vi "__PW_1ch.vi"(6 "Wait(ms)":i32=800, 8 "Ch（A,B,C,D）":string="A", 9 "A(A)":dbl=0.9, 10 "V(V)":dbl, 11 "GPIB":string="3") -> (1 "Amoni":dbl, 2 "Vmoni":dbl=0.05)   [LabVIEW 2017]
panel:
  out "文字列":string="VA0.00,AA0.90"
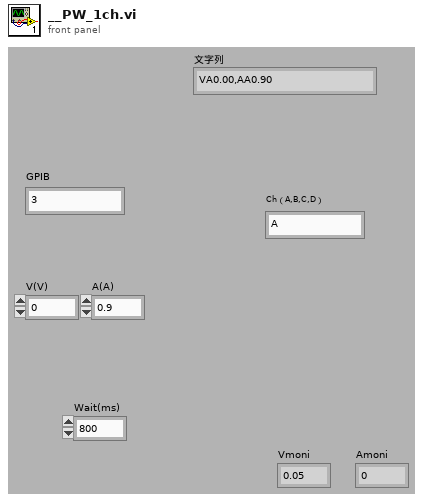
[diagram p1: front panel]
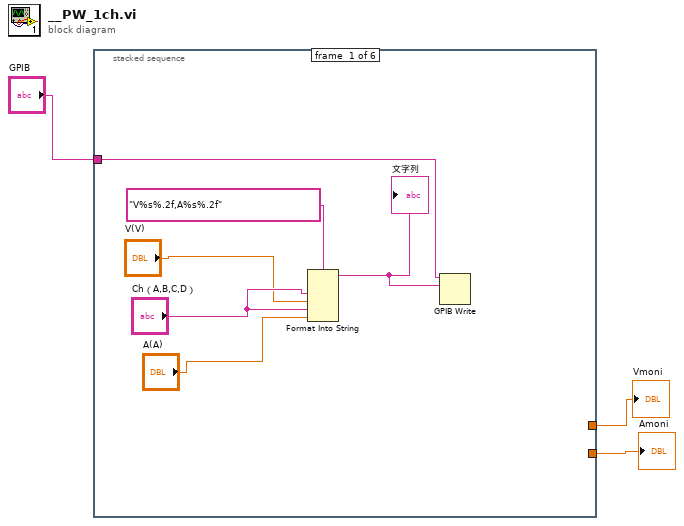
[diagram p0: block diagram]
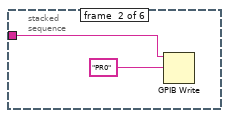
[diagram p2: hidden frame]
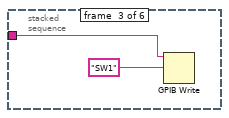
[diagram p3: hidden frame]
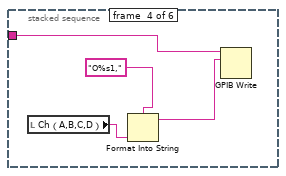
[diagram p4: hidden frame]
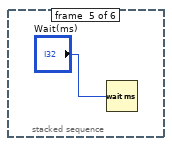
[diagram p5: hidden frame]
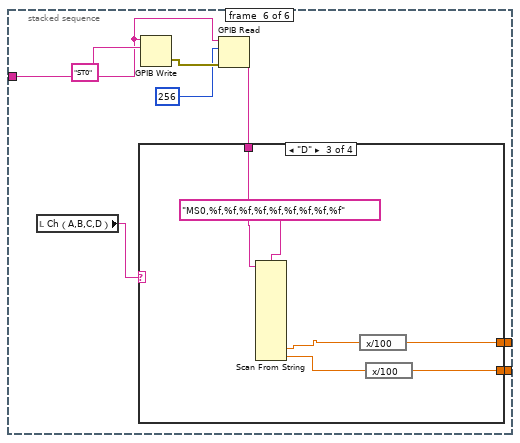
[diagram p6: hidden frame]
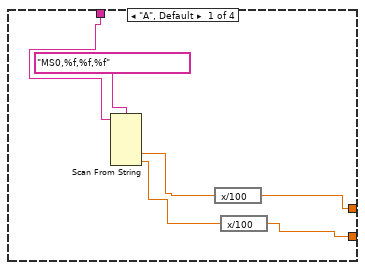
[diagram p7: hidden frame]
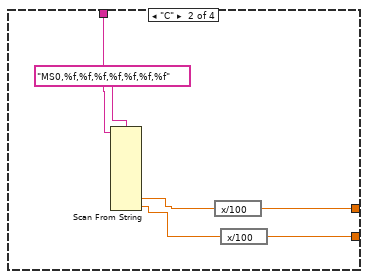
[diagram p8: hidden frame]
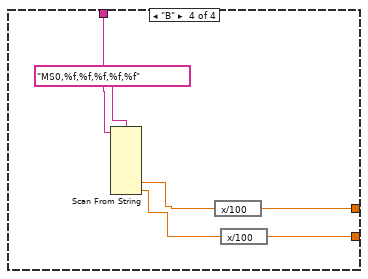
[diagram p9: hidden frame]
diagram:
  n1 = stacked-sequence {
    tunnel: "GPIB" -> [w8 w11 w13 w17 _ w24]
    tunnel: [_ _ _ _ _ w20] -> w2
    tunnel: [_ _ _ _ _ w19] -> w1
    frame #0 {
      n2 = Format Into String(format string="V%s%.2f,A%s%.2f", "Ch（A,B,C,D）", "V(V)", "Ch（A,B,C,D）", "A(A)") -> (resulting string=w7:string)  [unwired: 2 in, 1 out]
      "文字列" <- w7
      n3 = GPIB Write(0:w8, 1:w7) -> ()  [unwired: 3 in, 2 out]
    }
    frame #1 {
      n4 = GPIB Write(0:w11, 1:"PR0") -> ()  [unwired: 3 in, 2 out]
    }
    frame #2 {
      n5 = GPIB Write(0:w13, 1:"SW1") -> ()  [unwired: 3 in, 2 out]
    }
    frame #3 {
      n6 = local read "Ch（A,B,C,D）"() -> (w15:string)
      n7 = Format Into String(format string="O%s1,", w15) -> (resulting string=w14:string)  [unwired: 2 in, 1 out]
      n8 = GPIB Write(0:w17, 1:w14) -> ()  [unwired: 3 in, 2 out]
    }
    frame #4 {
      n9 = Wait (ms)(milliseconds to wait="Wait(ms)") -> ()  [unwired: 1 out]
    }
    frame #5 {
      n10 = local read "Ch（A,B,C,D）"() -> (w21:string)
      n11 = GPIB Write(0:w24, 1:"ST0") -> (6:w25:errorcluster)  [unwired: 3 in, 1 out]
      n12 = GPIB Read(0:w24, 1:256, 3:w25) -> (5:w22:string)  [unwired: 2 in, 2 out]
      n13 = case shown="\"D\"" w21 {
        tunnel: w22 -> [w31 w38 w44 w50]
        tunnel: [w28 w34 w42 w48] -> w20
        tunnel: [w27 w33 w41 w47] -> w19
        frame "A", Default {
          n14 = Scan From String(format string="MS0,%f,%f,%f", input string=w31) -> (output 2=w30:dbl, output 3=w29:dbl)  [unwired: 6 in, 3 out]
          n15 = expression code="x/100"(w30) -> (w28:dbl)
          n16 = expression code="x/100"(w29) -> (w27:dbl)
        }
        frame "C" {
          n17 = Scan From String(format string="MS0,%f,%f,%f,%f,%f,%f,%f", input string=w38) -> (output 6=w36:dbl, output 7=w35:dbl)  [unwired: 14 in, 3 out]
          n18 = expression code="x/100"(w36) -> (w34:dbl)
          n19 = expression code="x/100"(w35) -> (w33:dbl)
        }
        frame "D" {
          n20 = Scan From String(format string="MS0,%f,%f,%f,%f,%f,%f,%f,%f,%f", input string=w44) -> (output 8=w39:dbl, output 9=w40:dbl)  [unwired: 18 in, 3 out]
          n21 = expression code="x/100"(w39) -> (w42:dbl)
          n22 = expression code="x/100"(w40) -> (w41:dbl)
        }
        frame "B" {
          n23 = Scan From String(format string="MS0,%f,%f,%f,%f,%f", input string=w50) -> (output 4=w46:dbl, output 5=w45:dbl)  [unwired: 10 in, 3 out]
          n24 = expression code="x/100"(w46) -> (w48:dbl)
          n25 = expression code="x/100"(w45) -> (w47:dbl)
        }
      }
    }
  }
  "Vmoni" <- w2
  "Amoni" <- w1
